vi "Write Data.vi"(6 "NoStop (F)":bool, 7 "I2C Peripheral":refnum<class "I2C Peripheral.lvclass">, 8 "error in (no error)":errorcluster, 10 "Data":string) -> (0 "error out":errorcluster)   [LabVIEW 2020, in "CTI.lvlib" / "I2C Peripheral.lvclass"]
uses:
  I2C Peripheral.lvclass
  I2C Peripheral.lvclass/I2C Peripheral.ctl
  Session/Session.lvclass
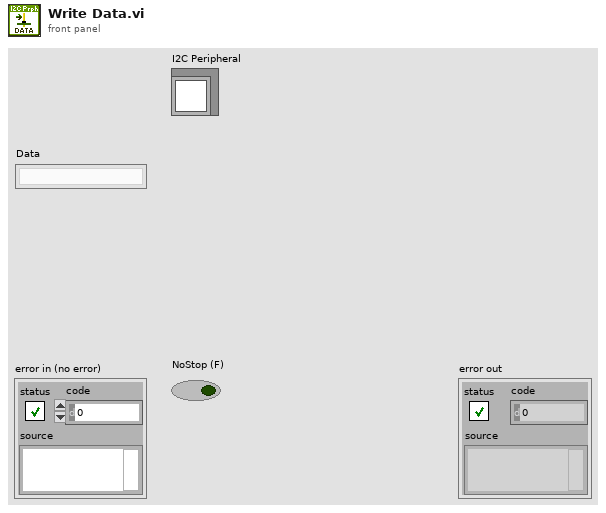
[diagram p1: front panel]
types:
  T1 = typedef "CTI.lvlib/I2C Address.ctl" = u8
  T2 = typedef "CTI.lvlib/I2C Number.ctl" = i8
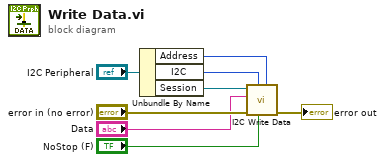
[diagram p0: block diagram]
diagram:
  n1 = Unbundle By Name("I2C Peripheral") -> ("Address"=w4:T1, "I2C"=w5:T2, "Session"=w1:refnum<class "Session.lvclass">)
  n2 = call "I2C Write Data.vi"("Address"=w4, "NoStop (F)"="NoStop (F)", "I2C #"=w5, "error in (no error)"="error in (no error)", "Data"="Data", "Session in"=w1) -> ("error out"=→"error out":errorcluster)  [unwired: 4 in, 1 out]
